vi "PhotonCamera_GetLEDMode.vi"() -> (0 "error out":errorcluster, 3 "LEDMode":T1)   [LabVIEW 2019, in "PhotonVisionLib.lvlib"]
doc: "Returns the current LED mode.\n\nInputs:\n <none>\n\nOutputs:\n - LedMode -- The current LED mode."
uses:
  PhotonVisionLib.lvlib
  Enum/VisionLEDModeType.ctl
  <vilib>/Rock Robotics/Network Tables/NT Read Integer.vi
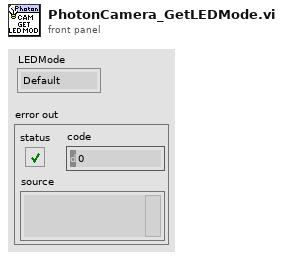
[diagram p1: front panel]
types:
  T1 = typedef "PhotonVisionLib.lvlib/VisionLEDModeType.ctl" = enum16{"Default", "Off", "On", "Blink"}
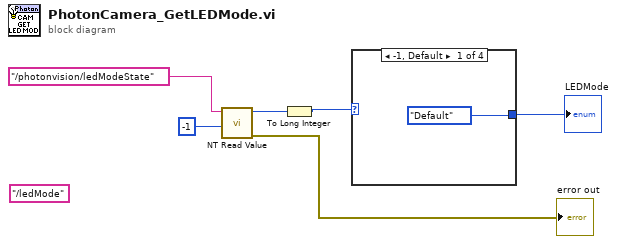
[diagram p0: block diagram]
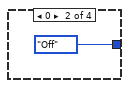
[diagram p2: hidden frame]
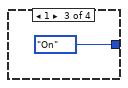
[diagram p3: hidden frame]
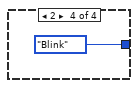
[diagram p4: hidden frame]
diagram:
  (unwired) "/ledMode"
  n1 = call-poly <vilib>:"NT Read Value.vi"("default value"=i64 -1 ("Default Value"), "name"="/photonvision/ledModeState") -> ("error out"=→"error out":errorcluster, "value"=w5:i64)  [unwired: 7 in, 1 out]
  n2 = To Long Integer(number=w5) -> (32bit integer=w4:i32)
  n3 = case shown="-1, Default" w4 {
    tunnel: [VisionLEDModeType."Default" ("LEDMode") VisionLEDModeType."Off" ("LEDMode") VisionLEDModeType."On" ("LEDMode") VisionLEDModeType."Blink" ("LEDMode")] -> w3
    frame -1, Default {
    }
    frame 0 {
    }
    frame 1 {
    }
    frame 2 {
    }
  }
  "LEDMode" <- w3
